vi "MotorMove.vi"(0 "Left Enc. Distance":dbl, 1 "Right Enc. Distance":dbl, 2 "Left Desired":dbl, 3 "Right Desired":dbl) -> ()   [LabVIEW 2014]
uses:
  Robot Global Data.vi
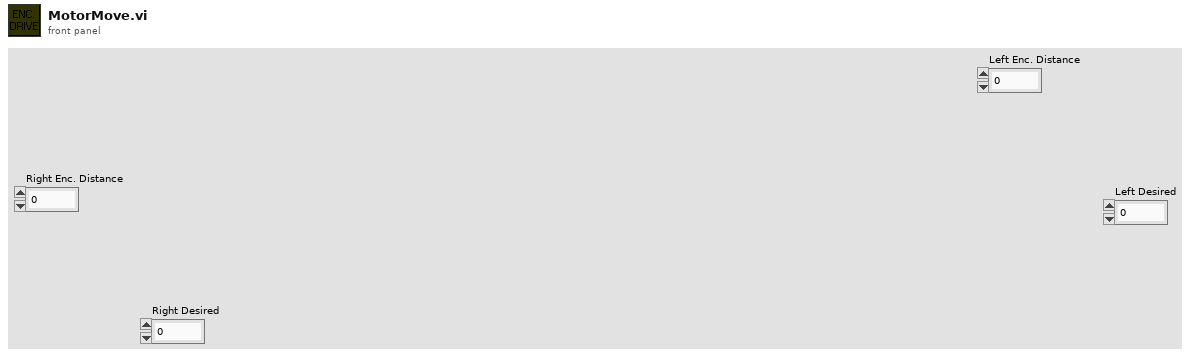
[diagram p1: front panel]
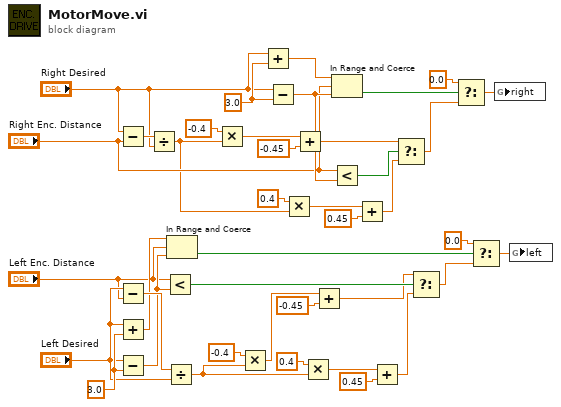
[diagram p0: block diagram]
diagram:
  w6 = 3.0 ("y")
  w39 = 3.0 ("y")
  n1 = Subtract(x="Right Desired", y="Right Enc. Distance") -> (x-y=w31:dbl)
  n2 = Subtract(x="Left Desired", y="Left Enc. Distance") -> (x-y=w12:dbl)
  n3 = Add(x="Left Desired", y=w6) -> (x+y=w5:dbl)
  n4 = Subtract(x="Left Desired", y=w6) -> (x-y=w9:dbl)
  n5 = Divide(x=w31, y="Right Desired") -> (x/y=w27:dbl)
  n6 = Less?(x="Left Enc. Distance", y=w9) -> (x < y?=w11:bool)
  n7 = Divide(x=w12, y="Left Desired") -> (x/y=w15:dbl)
  n8 = In Range and Coerce(upper limit=w5, x="Left Enc. Distance", lower limit=w9) -> (In Range?=w7:bool)  [unwired: 1 out]
  n9 = Multiply(x=-0.4 ("f"), y=w27) -> (x*y=w22:dbl)
  n10 = Multiply(x=-0.4 ("f"), y=w15) -> (x*y=w20:dbl)
  n11 = Add(x="Right Desired", y=w39) -> (x+y=w40:dbl)
  n12 = Subtract(x="Right Desired", y=w39) -> (x-y=w36:dbl)
  n13 = Multiply(x=0.4 ("t"), y=w27) -> (x*y=w26:dbl)
  n14 = Add(x=w22, y=-0.45) -> (x+y=w21:dbl)
  n15 = Multiply(x=0.4 ("t"), y=w15) -> (x*y=w16:dbl)
  n16 = Add(x=w20, y=-0.45) -> (x+y=w2:dbl)
  n17 = In Range and Coerce(upper limit=w40, x="Right Enc. Distance", lower limit=w36) -> (In Range?=w38:bool)  [unwired: 1 out]
  n18 = Less?(x="Right Enc. Distance", y=w36) -> (x < y?=w33:bool)
  n19 = Add(x=w26, y=0.45) -> (x+y=w24:dbl)
  n20 = Add(x=w16, y=0.45) -> (x+y=w18:dbl)
  n21 = Select(t=w21, s=w33, f=w24) -> (s? t:f=w35:dbl)
  n22 = Select(t=w2, s=w11, f=w18) -> (s? t:f=w10:dbl)
  n23 = Select(t=0.0, s=w38, f=w35) -> (s? t:f=w34:dbl)
  n24 = Select(t=0.0, s=w7, f=w10) -> (s? t:f=w1:dbl)
  n25 = global write "Robot Global Data.vi" "right"(w34) -> ()
  n26 = global write "Robot Global Data.vi" "left"(w1) -> ()
